vi "Display.vi"(8 "error in (no error)":errorcluster, 10 "ImageIndex":i32, 11 "ImageOperation in":refnum<class "ImageOperation.lvclass">) -> (0 "error out":errorcluster, 2 "Image Out":T1, 3 "ImageOperation out":refnum<class "ImageOperation.lvclass">)   [LabVIEW 2015, in "ImageOperation.lvclass"]
uses:
  ImageOperation.lvclass
  <vilib>/vision/Image Controls.llb/IMAQ Image.ctl
  ImageOperation.lvclass/ImageOperation.ctl
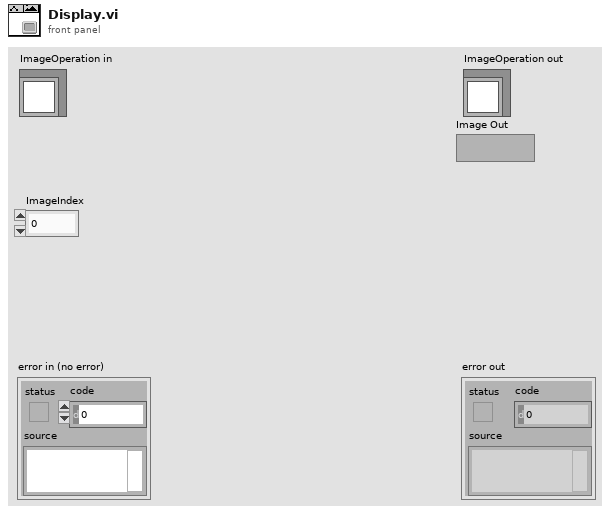
[diagram p1: front panel]
types:
  T1 = typedef "IMAQ Image.ctl" = refnum<image>
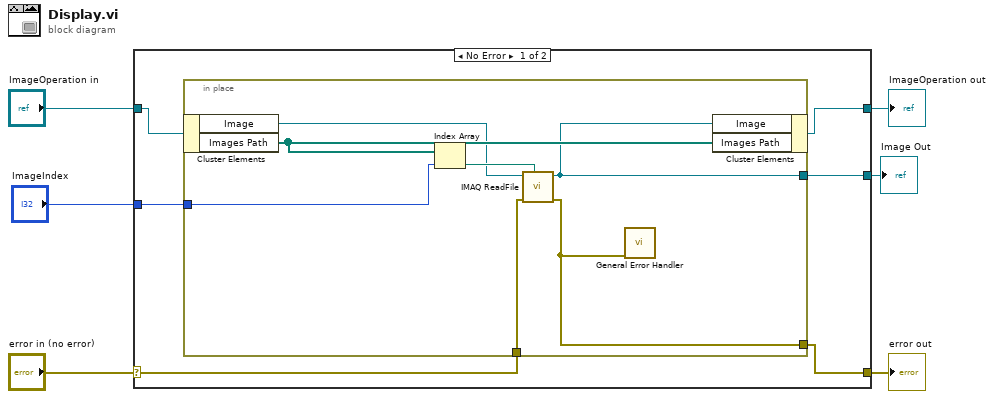
[diagram p0: block diagram]
diagram:
  n1 = case shown="No Error" "error in (no error)" {
    selector: "error in (no error)" -> [w12 w21]
    tunnel: [w10 w21] -> w5
    tunnel: [w9 w20] -> w3
    tunnel: "ImageOperation in" -> [w11 w20]
    tunnel: "ImageIndex" -> [w8 _]
    tunnel: [w7 _] -> w1
    frame No Error {
      n2 = in-place {
        in-place-border: w12 -> [w19]
        in-place-border: [w13] -> w10
        in-place-border: w8 -> [w15]
        in-place-border: [w14] -> w7
        n3 = in-place-cluster #1(w11) -> ("Image"=w16:T1, "Images Path"=w17:path[])
        n4 = Index Array(array=w17, index=w15) -> (element=w18:path)
        n5 = call "IMAQ ReadFile"("File Path"=w18, "error in (no error)"=w19, "Image"=w16) -> ("error out"=w13:errorcluster, "Image Out"=w14:T1)  [unwired: 4 in, 3 out]
        n6 = call <vilib>:"General Error Handler.vi"("error in (no error)"=w13) -> ()  [unwired: 10 in, 5 out]
        n7 = in-place-cluster #1("Image"=w14, "Images Path"=w17) -> (w9:refnum<class "ImageOperation.lvclass">)
      }
    }
    frame Error {
    }
  }
  "error out" <- w5
  "ImageOperation out" <- w3
  "Image Out" <- w1
